vi "StopVI.vi"(0 "Application Ref in":refnum<vi>, 5 "VI in":refnum<vi>, 11 "error in (no error)":errorcluster) -> (15 "error out":errorcluster)   [LabVIEW 2016, in "CarWashTest.lvlib"]
doc: "Stop the main VI"
uses:
  CarWashTest.lvlib
  APIs/Stimulus/VI/OpenVIFrontPanel.vi
  APIs/Stimulus/ControlValue/ValueSignalLatchBooleanString.vi
  Drona.lvlib
  APIs/Stimulus/VI/VI.lvlib
  APIs/Stimulus/ControlValue/ControlValue.lvlib
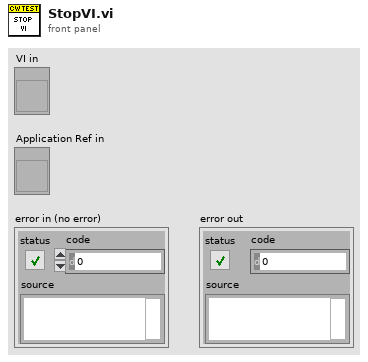
[diagram p1: front panel]
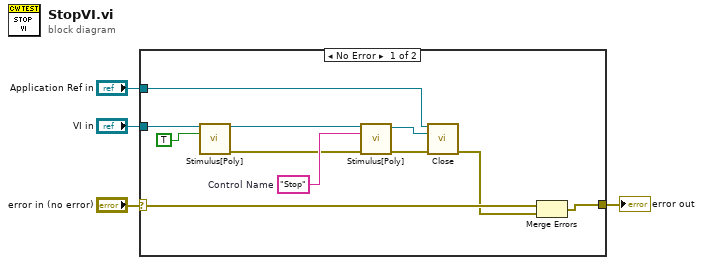
[diagram p0: block diagram]
diagram:
  n1 = case shown="No Error" "error in (no error)" {
    selector: "error in (no error)" -> [w15 w16]
    tunnel: [w14 w16] -> w3
    tunnel: "VI in" -> [w10 _]
    tunnel: "Application Ref in" -> [w8 _]
    frame No Error {
      w13 = "Stop"  # Control Name
      n2 = call-poly "Stimulus[Poly].vi"("VI Reference In"=w10, "Activate (F)"=TRUE ("Wait Until Done (F)")) -> ("VI Reference Out"=w11:refnum<vi>, "error out"=w9:errorcluster)  [unwired: 12 in]
      n3 = call-poly "Stimulus[Poly].vi"("VI Reference In"=w11, "Control Path"=w13, "error in"=w9) -> ("VI Reference Out"=w7:refnum<vi>, "error out"=w6:errorcluster)  [unwired: 11 in]
      n4 = call "Close.vi"("Application Ref"=w8, "VI Reference"=w7, "error in"=w6) -> ("error out"=w5:errorcluster)  [unwired: 12 in]
      n5 = Merge Errors(w15, w5) -> (w14:errorcluster)
    }
    frame Error {
    }
  }
  "error out" <- w3
